vi "Firmware 3 - Mauricio Oro Natel.vi"() -> ()   [LabVIEW 2017]
uses:
  <vilib>/LabVIEW Interface for Arduino/Type Defs/Pin Mode.ctl
  <vilib>/LabVIEW Interface for Arduino/Type Defs/Board Type.ctl
  <vilib>/LabVIEW Interface for Arduino/Type Defs/Connection Type.ctl
  <vilib>/LabVIEW Interface for Arduino/LabVIEW Interface for Arduino.lvlib
panel:
  out "Atuador S1":bool
  in  "Fora de Padrão":bool
  in  "VISA resource":refnum<visa-resource-name>
  out "Fora de Padrão":bool
  in  "Peça Baixa":bool
  out "Esteira":bool
  in  "Peça Alta/Baixa":bool
  in  "Liga":bool
  in  "stop":bool
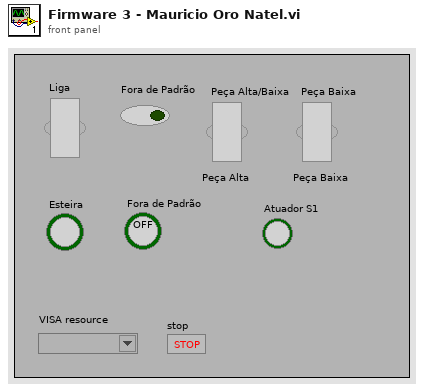
[diagram p1: front panel]
types:
  T1 = typedef "LabVIEW Interface for Arduino.lvlib/Connection Type.ctl" = enum8{"USB / Serial", "XBEE", "BlueSmirf (Bluetooth)"}
  T2 = typedef "LabVIEW Interface for Arduino.lvlib/Board Type.ctl" = enum16{"Uno", "Dimuelanove w/Atmega 328", "Mega 2560"}
  T3 = typedef "LabVIEW Interface for Arduino.lvlib/Pin Mode.ctl" = enum8{"Input", "Output"}
  T4 = typedef "LabVIEW Interface for Arduino.lvlib/Arduino Resource.ctl" = cluster{"VISA resource":refnum<visa-resource-name>, "Board Type":T2, "Connection Type":enum8{"USB / Serial"}, "Bytes Per Packet (15)":u8}
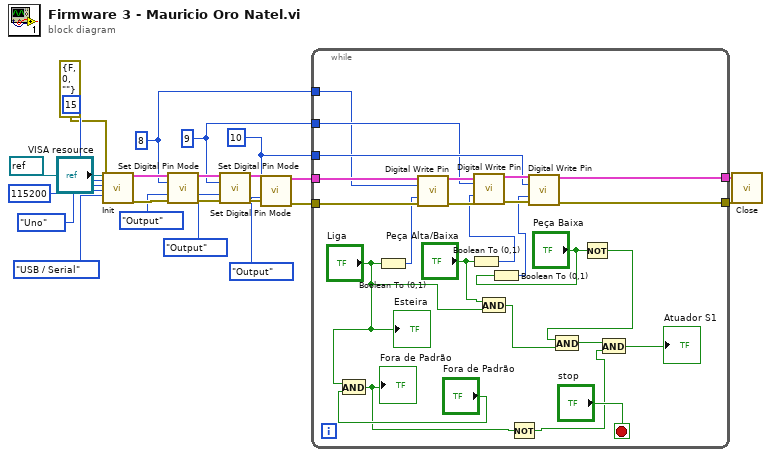
[diagram p0: block diagram]
diagram:
  w5 = u8 10 ("Digital I/O Pin")
  w4 = u8 9 ("Digital I/O Pin")
  w3 = u8 8 ("Digital I/O Pin")
  n1 = call <vilib>:"Init.vi"("VISA resource"=refnum<visa-resource-name> refnum, "Baud Rate (115200)"=u32 115200, "Board Type (Uno)"=Board_Type."Uno", "Bytes Per Packet (15)"=u32 15, "Connection Type (USB/Serial)"=Connection_Type."USB / Serial", "error in"=errorcluster {"status"=FALSE, "code"=0, "source"=""}) -> ("Arduino Resource"=w22:T4, "error out"=w21:errorcluster)  [unwired: 12 in]
  n2 = call <vilib>:"Set Digital Pin Mode.vi"("Arduino Resource"=w22, "Digital I/O Pin"=w3, "Pin Mode (Input)"=Pin_Mode."Output", "error in"=w21) -> ("Arduino Resource"=w20:T4, "error out"=w18:errorcluster)  [unwired: 10 in]
  n3 = call <vilib>:"Set Digital Pin Mode.vi"("Arduino Resource"=w20, "Digital I/O Pin"=w4, "Pin Mode (Input)"=Pin_Mode."Output", "error in"=w18) -> ("Arduino Resource"=w19:T4, "error out"=w17:errorcluster)  [unwired: 10 in]
  n4 = call <vilib>:"Set Digital Pin Mode.vi"("Arduino Resource"=w19, "Digital I/O Pin"=w5, "Pin Mode (Input)"=Pin_Mode."Output", "error in"=w17) -> ("Arduino Resource"=w16:T4, "error out"=w15:errorcluster)  [unwired: 10 in]
  n5 = while {
    tunnel: w16 -> [w47]
    tunnel: w15 -> [w44]
    tunnel: w5 -> [w41]
    tunnel: w4 -> [w40]
    tunnel: w3 -> [w39]
    tunnel: [w35] -> w2
    tunnel: [w34] -> w1
    stop <- "stop" stop-if-true
    n6 = And(x="Liga", y="Fora de Padrão") -> (x .and. y?=w23:bool)
    "Fora de Padrão" <- w23
    n7 = Boolean To (0,1)(Boolean="Liga") -> (0, 1=w37:i16)
    n8 = call <vilib>:"Digital Write Pin.vi"("Arduino Resource"=w47, "Digital I/O Pin (0)"=w39, "Value (0)"=w37, "error in"=w44) -> ("Arduino Resource"=w46:T4, "error out"=w43:errorcluster)  [unwired: 10 in]
    n9 = Boolean To (0,1)(Boolean="Peça Alta/Baixa") -> (0, 1=w36:i16)
    n10 = call <vilib>:"Digital Write Pin.vi"("Arduino Resource"=w46, "Digital I/O Pin (0)"=w40, "Value (0)"=w36, "error in"=w43) -> ("Arduino Resource"=w45:T4, "error out"=w42:errorcluster)  [unwired: 10 in]
    n11 = And(x="Peça Alta/Baixa", y="Liga") -> (x .and. y?=w28:bool)
    n12 = Boolean To (0,1)(Boolean="Peça Baixa") -> (0, 1=w33:i16)
    n13 = Not(x=w23) -> (.not. x?=w24:bool)
    n14 = call <vilib>:"Digital Write Pin.vi"("Arduino Resource"=w45, "Digital I/O Pin (0)"=w41, "Value (0)"=w33, "error in"=w42) -> ("Arduino Resource"=w35:T4, "error out"=w34:errorcluster)  [unwired: 10 in]
    n15 = Not(x="Peça Baixa") -> (.not. x?=w31:bool)
    n16 = And(x=w31, y=w28) -> (x .and. y?=w27:bool)
    n17 = And(x=w27, y=w24) -> (x .and. y?=→"Atuador S1":bool)
    "Esteira" <- "Liga"
  }
  n18 = call <vilib>:"Close.vi"("Arduino Resource"=w2, "error in"=w1) -> ()  [unwired: 13 in, 1 out]
